vi "Get Chamber ID.vi"() -> (3 "Current Chamber #":sgl, 5 "Current Chamber # (enum)":T1=enum."CH ABI", 6 "Chamber name":string)   [LabVIEW 2020]
doc: "This VI calls MACaddress.dll to get the first MAC address of the current computer, and compare it with the MAC addresses of the chambers set by the user.\nTo get MAC address in Windows:\nGo to Start->run, type in \"cmd\", a console window will pop up. Then type \"ipconfig/all\", the information after \"Physical Address\" is the MAC address . Copy that number and please remember to REMOVE THE DASHES.\n-- 12/2004 Haobing Wang"
uses:
  Chamber ID Enum.ctl
  Comparison VIs/Arrays Equal (U8).vi
  MACaddress.dll
panel:
  in  "Chamber List":cluster{"Chamber #":T1, "MAC address":u8[]}[](array[cluster])=[{"Chamber #"=enum."CH 4", "MAC address"=[0, 176, 208, 243, 168, 132]}, {"Chamber #"=enum."CH 1", "MAC address"=[0, 6, 91, 135, 165, 202]}, {"Chamber #"=enum."CH 411", "MAC address"=[0, 6, 91, 135, 94, 153]}, {"Chamber #"=enum."CH 412", "MAC address"=[0, 18, 63, 51, 216, 245]}, {"Chamber #"=enum."CH1-PXI", "MAC address"=[0, 128, 47, 16, 235, 96]}, {"Chamber #"=enum."CH ABI", "MAC address"=[0, 128, 47, 16, 187, 172]}, {"Chamber #"=enum."Puccini", "MAC address"=[0, 128, 47, 17, 228, 2]}, {"Chamber #"=enum."Bach", "MAC address"=[0, 128, 47, 17, 227, 244]}] {"MAC address" format="%x"}
  out "MAC address of the current computer":u8[](array[numeric])=[0, 128, 47, 16, 187, 172] format="%x"
  # "This VI calls MACaddress.dll to get the first MAC address  of the current computer, and compares it with the MAC addresses of the chambers set by the user here on the front panel.\n\nTo get MAC address in Windows:\nGo to Start->run, type in \"cmd\", a console window will pop up. Then type \"ipconfig/all\", the information after \"Physical Address\" is the MAC address . Copy that number and please remember to REMOVE THE DASHES.\n\n-- 12/2004 Haobing Wang"
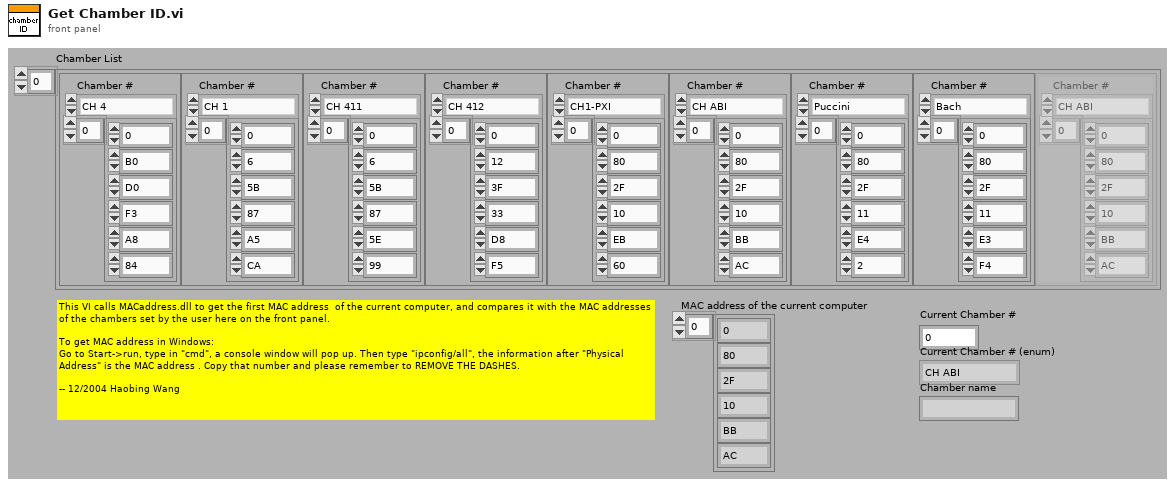
[diagram p1: front panel]
types:
  T1 = typedef "Chamber ID Enum.ctl" = enum16{"Unknown", "CH 1", "CH 4", "CH 411", "CH 412", "CH1-PXI", "CH ABI", "Puccini", "Bach"}
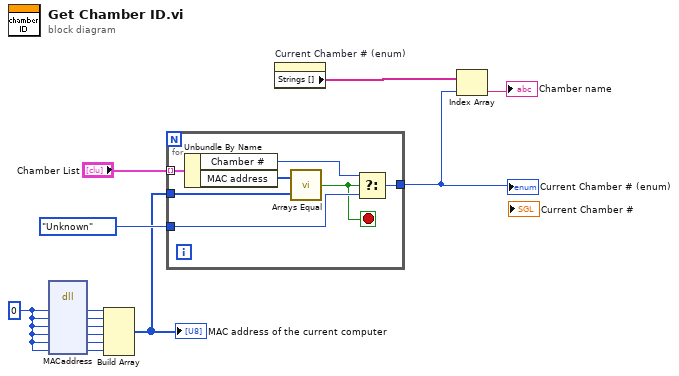
[diagram p0: block diagram]
diagram:
  w13 = u8 0 ("input param")
  n1 = dll-call lib="D:/Experiment VIs/Utility VIs/System Info VIs/MACaddress.dll" fn="MACaddress"(w13, w13, w13, w13, w13, w13) -> (w12:u8, w11:u8, w10:u8, w9:u8, w8:u8, w7:u8)  [unwired: 4 in, 2 out]
  n2 = Build Array(w12, w11, w10, w9, w8, w7) -> (w1:u8[])
  "MAC address of the current computer" <- w1
  n3 = for {
    tunnel: "Chamber List" -> [w20] mode=indexing
    tunnel: [w17] -> w2
    tunnel: Chamber_ID_Enum."Unknown" ("Current Chamber # (enum)") -> [w16]
    tunnel: w1 -> [w15]
    stop <- w14 stop-if-true
    n4 = Unbundle By Name(w20) -> ("Chamber #"=w18:T1, "MAC address"=w19:u8[])
    n5 = call-poly "Arrays Equal.vi"("Array 2"=w15, "Array 1"=w19) -> ("arrays equal?"=w14:bool)
    n6 = Select(t=w18, s=w14, f=w16) -> (s? t:f=w17:T1)
  }
  "Current Chamber # (enum)" <- w2
  n7 = property on="Current Chamber # (enum)" class="Enum (strict)"() -> ("Strings []"=w6:string[])  [unwired: 2 in, 2 out]
  n8 = Index Array(array=w6, index=w2) -> (element=→"Chamber name":string)
